vi "SSH_ReadWrite.vi"(6 "Timeout (ms)":u32, 8 "error in (no error)":errorcluster, 9 "Wait for":string, 10 "To Send":string, 11 "Python":T1) -> (0 "error out":errorcluster, 1 "Console":string)   [LabVIEW 2021]
uses:
  PythonCtrl.ctl
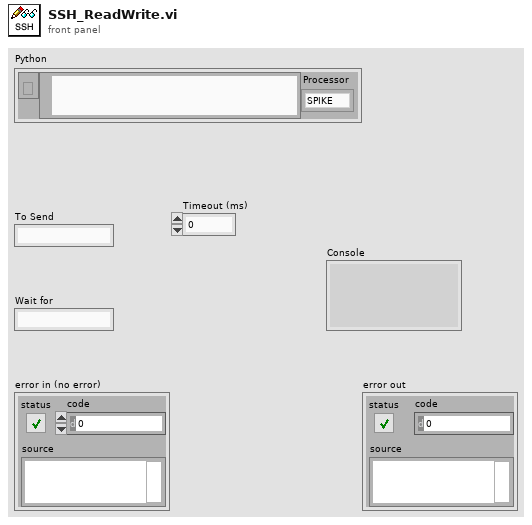
[diagram p1: front panel]
types:
  T1 = typedef "PythonCtrl.ctl" = cluster{"session":refnum<k35>, "PyPath":path, "Processor":enum16{"SPIKE", "Pi", "Pi_ssh"}}
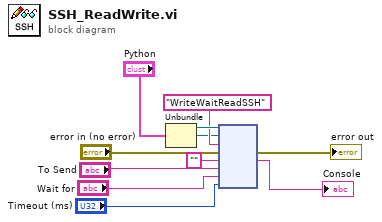
[diagram p0: block diagram]
diagram:
  n1 = Unbundle("Python") -> ("session"=w11:refnum<k35>, "PyPath"=w2:path)  [unwired: 1 out]
  n2 = node(w11, w2, "WriteWaitReadSSH" ("function name"), "error in (no error)", "" ("function name"), "To Send", "Wait for", "Timeout (ms)") -> (→"error out":errorcluster, →"Console":string)  [unwired: 3 in, 3 out]
